vi "RSNRPZ Set Sampling Frequency.vi"(8 "error in (no error)":errorcluster, 9 "Sampling Frequency (1: Sampling Frq 1 (High))":i32(ring)=1 items=["Sampling Frq 1 (High)"=1, "Sampling Frq 2 (Low)"=2], 10 "Channel (1)":i32=1, 11 "VISA session":refnum<visa-resource-name> caption="VISA resource name") -> (0 "error out":errorcluster, 3 "dup VISA session":refnum<visa-resource-name> caption="VISA resource name")   [LabVIEW 2010]
doc: "If the signal to be measured has modulation sections just above the video bandwidth of the sensor used, measurement errors might be caused due to aliasing effects. In this case, the sampling rate of the sensor can be set to a safe lower value (Sampling Frequency 2). However, the measurement time required to obtain noise-free results is extended compared to the normal sampling rate (Sampling Frequency 1).\n\nNote:\n\n1) This VI is not available for NRP-Z51.\n\nRemote-control command(s):\nSENS:SAMP FREQ1 | FREQ2"
uses:
  rsnrpz_32.dll
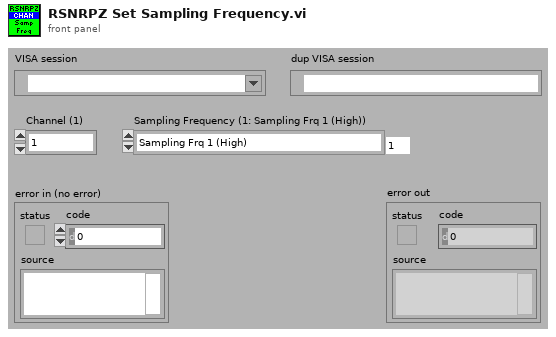
[diagram p1: front panel]
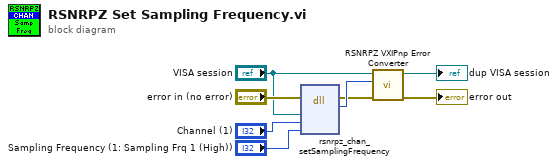
[diagram p0: block diagram]
diagram:
  n1 = dll-call lib="rsnrpz_32.dll" fn="rsnrpz_chan_setSamplingFrequency"(error in="error in (no error)", "VISA Session"="VISA session", "Channel"="Channel (1)", "Sampling Frequency"="Sampling Frequency (1: Sampling Frq 1 (High))") -> (error out=w5:errorcluster, "Status"=w8:i32)  [unwired: 5 in, 1 out]
  n2 = call <instrlib>:"RSNRPZ VXIPnp Error Converter.vi"("error in"=w5, "VXIPnp error code"=w8, "VISA session"="VISA session") -> ("error out"=→"error out":errorcluster, "dup VISA session"=→"dup VISA session":refnum<visa-resource-name>)  [unwired: 7 in]
